vi "jMsg_TCPConnection_Update - Rx Read.vi"(8 "error in (no error)":errorcluster, 11 "jModule":refnum<class "jModule.lvclass">) -> (0 "error out":errorcluster, 2 "Connection":T1, 3 "jModule":refnum<class "jModule.lvclass">, 7 "jMsg_TCPConnection_Update":refnum<class "jMsg_TCPConnection_Update.lvclass">)   [LabVIEW 2019, in "jMsg_TCPConnection_Update.lvclass"]
doc: "This VI is used to read data from the jMsg\n\n\nJSMA Message Wizard 0.2.0.5\nRob Humfeld - Jet Engineering\nCopyright (c) 2020, Jet Engineering"
uses:
  jMsg_TCPConnection_Update.lvclass
  <userlib>/Jet Engineering/JSMA/Libraries/jModule Class/jModule.lvclass
  TCPConnectionSettings STYP.ctl
  <userlib>/Jet Engineering/JSMA/Libraries/jModule Class/jModule.lvclass/jModule.ctl
  jMsg_TCPConnection_Update.lvclass/jMsg_TCPConnection_Update.ctl
panel:
  in  "jMsg_TCPConnection_Update":refnum<class "jMsg_TCPConnection_Update.lvclass">
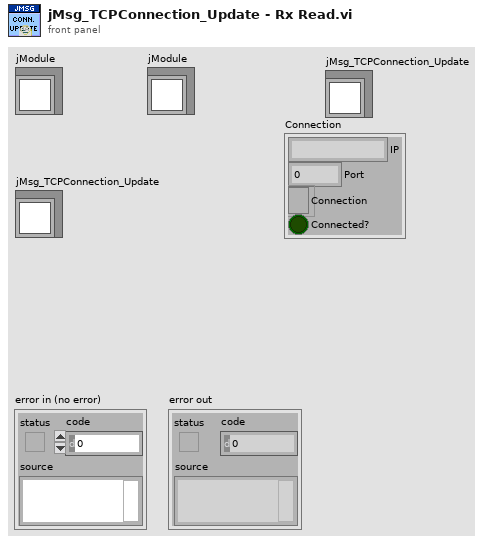
[diagram p1: front panel]
types:
  T1 = typedef "TCPConnectionSettings STYP.ctl" = cluster{"IP":string, "Port":u32, "Connection":refnum<k5>, "Connected?":bool}
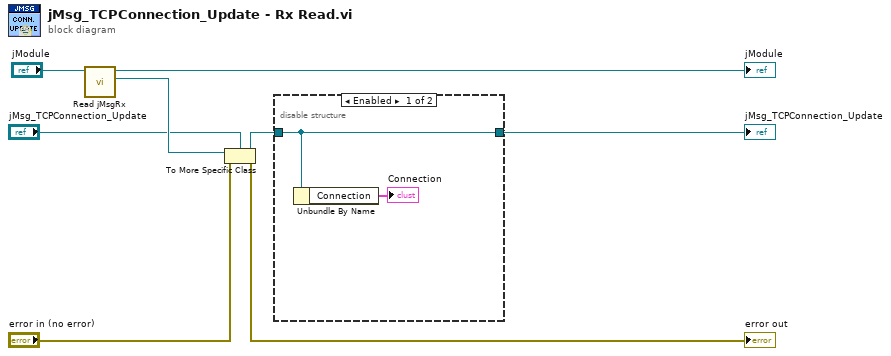
[diagram p0: block diagram]
diagram:
  n1 = call <userlib>:"Read jMsgRx.vi"("jModule in"="jModule") -> ("Received jMsg"=w5:refnum<class "jMsg.lvclass">, "jModule out"=→"jModule":refnum<class "jModule.lvclass">)  [unwired: 8 in, 1 out]
  n2 = To More Specific Class(target class="jMsg_TCPConnection_Update", reference=w5, error in="error in (no error)") -> (specific class reference=w3:refnum<class "jMsg_TCPConnection_Update.lvclass">, error out=→"error out":errorcluster)
  n3 = disable-structure shown="Enabled" {
    disable-tunnel: w3 -> [w10 w11]
    disable-tunnel: [w10 w11] -> w8
    frame Enabled {
      n4 = Unbundle By Name(w10) -> ("Connection"=→"Connection":T1)
    }
    frame Disabled {
    }
  }
  "jMsg_TCPConnection_Update" <- w8
